vi "High g status decoder.vi"(0 "Force NA(F)":bool, 7 "High G Code":u8 format="%08b") -> (4 "Monitoring":T1, 6 "Recording":T1, 8 "Data ready":T1, 14 "Array (monitor, Record,, data ready)":T1[](array[typedef]))   [LabVIEW 2011]
uses:
  Measurments Handling/Status Digitalish.ctl
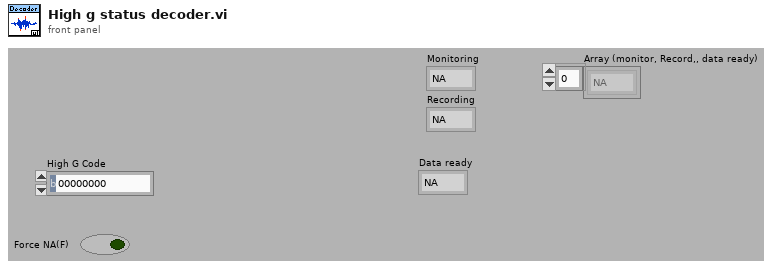
[diagram p1: front panel]
types:
  T1 = typedef "Status Digitalish.ctl" = enum16{"NA", "False", "True"}
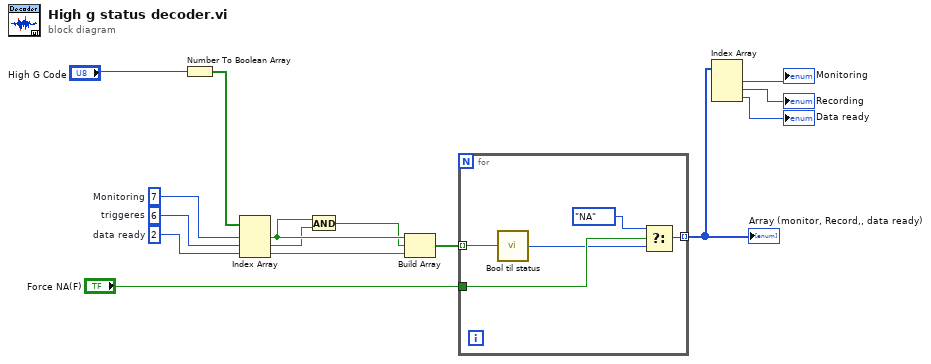
[diagram p0: block diagram]
diagram:
  w5 = 2  # data ready
  w6 = 6  # triggeres
  w7 = 7  # Monitoring
  n1 = Number To Boolean Array(number="High G Code") -> (Boolean array=w8:bool[])
  n2 = Index Array(array=w8, index #1=w7, index #2=w6, index #3=w5) -> (element #1=w3:bool, element #2=w2:bool, element #3=w4:bool)
  n3 = And(x=w3, y=w2) -> (x .and. y?=w1:bool)
  n4 = Build Array(w3, w1, w4) -> (w11:bool[])
  n5 = for {
    tunnel: w11 -> [w17] mode=indexing
    tunnel: [w20] -> w10 mode=indexing
    tunnel: "Force NA(F)" -> [w19]
    n6 = call "Bool til status.vi"("Boolean"=w17) -> ("Status"=w16:T1)  [unwired: 8 in]
    n7 = Select(t=Status_Digitalish."NA" ("Monitoring"), s=w19, f=w16) -> (s? t:f=w20:T1)
  }
  "Array (monitor, Record,, data ready)" <- w10
  n8 = Index Array(array=w10) -> (element #1=→"Monitoring":T1, element #2=→"Recording":T1, element #3=→"Data ready":T1)  [unwired: 3 in]
